vi "zadanie_2.vi"() -> ()   [LabVIEW 2020]
uses:
  <vilib>/numeric/Random Number (Range) DBL.vi
  <vilib>/Analysis/NI_AALBase.lvlib
panel:
  out "XY Graph":cluster{"Y":dbl[], "Y":dbl[]}[](graph)
  out "mediana":dbl
  out "maksimum":dbl
  out "minimum":dbl
  in  "stop":bool
  in  "generuj":bool
  in  "maks":dbl
  in  "min":dbl
  in  "liczba losowan":dbl
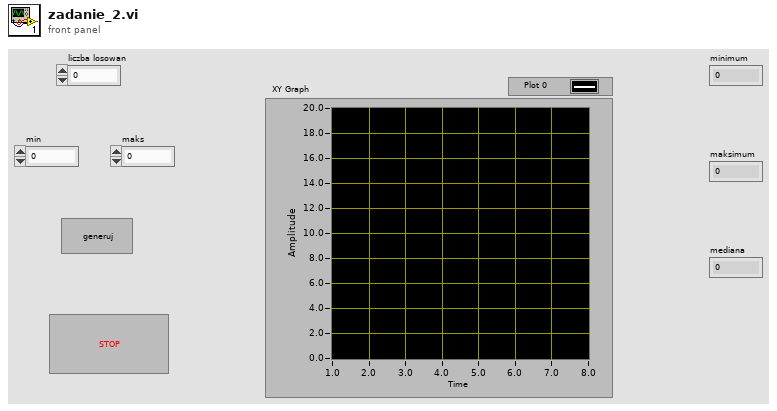
[diagram p1: front panel]
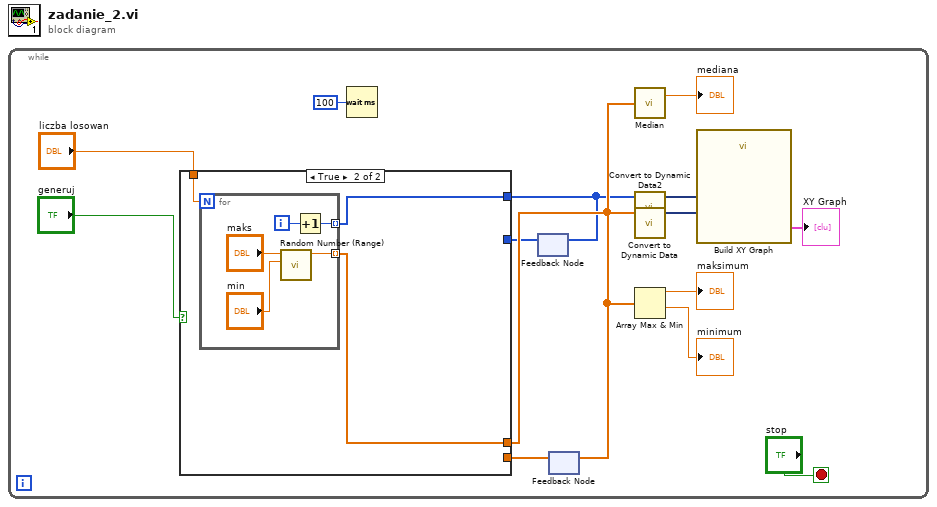
[diagram p0: block diagram]
diagram:
  n1 = while {
    stop <- "stop" stop-if-true
    n2 = Wait (ms)(milliseconds to wait=u32 100) -> ()  [unwired: 1 out]
    n3 = feedback #1() -> (w1:i32[])  [unwired: 1 in]
    n4 = feedback #2() -> (w5:dbl[])  [unwired: 1 in]
    n5 = case shown="True" "generuj" {
      tunnel: "liczba losowan" -> [_ w19]
      tunnel: w5 -> [w16 _]
      tunnel: [w16 w18] -> w4
      tunnel: [w15 w17] -> w2
      tunnel: w1 -> [w15 _]
      frame False {
      }
      frame True {
        n6 = for {
          N: w19 -> [_]
          tunnel: [w22] -> w18 mode=indexing
          tunnel: [w20] -> w17 mode=indexing
          i -> [w21]
          n7 = call-poly <vilib>:"Random Number (Range).vi"("lower bound (0)"="min", "upper bound (100)"="maks") -> ("number"=w22:dbl)  [unwired: 9 in]
          n8 = Increment(x=w21) -> (x+1=w20:i32)
        }
      }
    }
    n9 = feedback-in #1(w2) -> ()
    n10 = feedback-in #2(w4) -> ()
    n11 = call <vilib>:"Median.vi"("X"=w4) -> ("median"=→"mediana":dbl)  [unwired: 1 out]
    n12 = call "Convert to Dynamic Data2"("Array"=w2) -> ("Dynamic Data Type"=w3:dynamicdata)  [unwired: 3 in]
    n13 = call "Convert to Dynamic Data"("Array"=w4) -> ("Dynamic Data Type"=w6:dynamicdata)  [unwired: 3 in]
    n14 = Array Max & Min(array=w4) -> (max value=→"maksimum":dbl, min value=→"minimum":dbl)  [unwired: 2 out]
    n15 = call "Build XY Graph"("Y Input"=w6, "X Input"=w3) -> ("XY Graph"=→"XY Graph":cluster{"X":dbl[], "Y":dbl[]}[])  [unwired: 8 in, 1 out]
  }
